vi "Lissajou.vi"() -> ()   [LabVIEW 2017]
panel:
  in  "stop":bool
  out "?":cluster{"Y":dbl[], "Y":dbl[]}[](graph)
  in  "Frequenz f2":dbl(slide) scale=0.0..400.0
  in  "Phase phi1":dbl(slide) scale=0.0..3.141592653589793
  in  "Frequenz f1":dbl(slide) scale=0.0..400.0
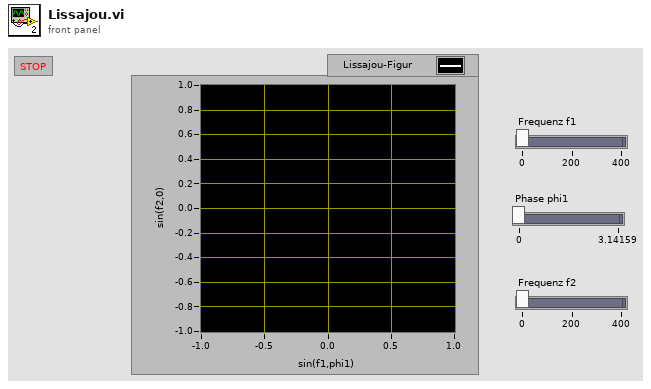
[diagram p1: front panel]
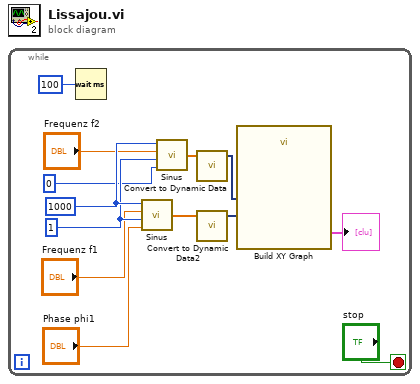
[diagram p0: block diagram]
diagram:
  n1 = while {
    stop <- "stop" stop-if-true
    w13 = 1000
    w12 = 1
    n2 = Wait (ms)(milliseconds to wait=100) -> ()  [unwired: 1 out]
    n3 = call "Sinus.vi"("Phase phi"="Phase phi1", "Amplitude A"=w12, "Frequenz f"="Frequenz f1", "Datenpunkte N"=w13) -> ("sin(t_i)"=w6:dbl[])
    n4 = call "Sinus.vi"("Phase phi"=0, "Amplitude A"=w12, "Frequenz f"="Frequenz f2", "Datenpunkte N"=w13) -> ("sin(t_i)"=w5:dbl[])
    n5 = call "Convert to Dynamic Data"("Array"=w5) -> ("Dynamic Data Type"=w3:dynamicdata)  [unwired: 3 in]
    n6 = call "Convert to Dynamic Data2"("Array"=w6) -> ("Dynamic Data Type"=w2:dynamicdata)  [unwired: 3 in]
    n7 = call "Build XY Graph"("Y Input"=w2, "X Input"=w3) -> ("XY Graph"=→"?":cluster{"X":dbl[], "Y":dbl[]}[])  [unwired: 8 in, 1 out]
  }
